vi "removeEmptyArrayElement.vi"(8 "error in (no error)":errorcluster, 10 "Array in":string[](array[string]), 11 "AttributeReader in":refnum<class "XMLAttributeParser.lvclass">) -> (0 "error out":errorcluster, 2 "Array out":string[](array[string]), 3 "AttributeReader out":refnum<class "XMLAttributeParser.lvclass">)   [LabVIEW 2014, in "XML.lvlib" / "XMLAttributeParser.lvclass"]
doc: "The parsing leaves behind an empty string as the last value of the array. This method cleans that up and is called when attributes are parsed into an array."
uses:
  <userlib>/Common/XML/XMLAttributeParser/XMLAttributeParser.lvclass
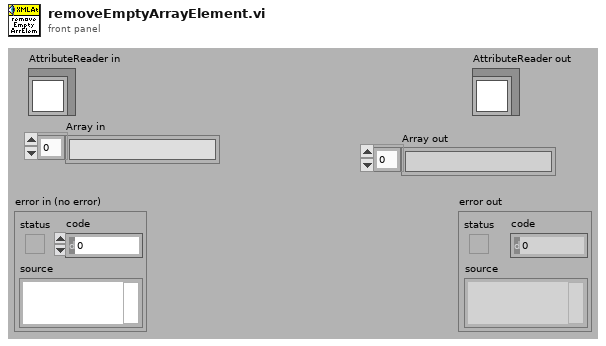
[diagram p1: front panel]
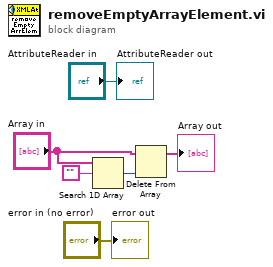
[diagram p0: block diagram]
diagram:
  n1 = Search 1D Array(1D array="Array in", element="") -> (index of element=w3:i32)  [unwired: 1 in]
  n2 = Delete From Array(array="Array in", index=w3) -> (array with subset deleted=→"Array out":string[])  [unwired: 1 in, 1 out]
  "AttributeReader out" <- "AttributeReader in"
  "error out" <- "error in (no error)"
